vi "info Handler LV.vi"(11 "instance":i32) -> ()   [LabVIEW 2022 SP3, in "SADI_FW3.lvlib"]
doc: "SADI_API_Wrapper void infoHandler_LV(int instance);"
uses:
  SADI_FW3.lvlib
  SADI_FW3.dll
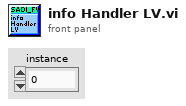
[diagram p1: front panel]
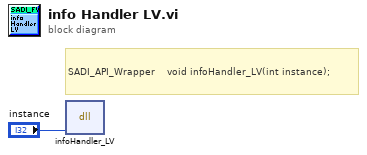
[diagram p0: block diagram]
diagram:
  # "SADI_API_Wrapper    void infoHandler_LV(int instance);"
  n1 = dll-call lib="C:/Users/scer/OneDrive - University of Florida/eml4314c/eml4314Sp24/Resources/release_1_11_24/EML4314c_Sp24_framework_0/LVLib/SADI_FW3.*" fn="infoHandler_LV"("instance"="instance") -> ()  [unwired: 5 in, 2 out]
